vi "PH_SRDG645.get data to modify.vi"(0 "i ref in":refnum<vi>, 3 "ms timeout (10000)":i32=10000, 5 "error in (no error)":errorcluster) -> (14 "i ref out":refnum<vi>, 16 "i attribute":T1={"GUI Refs"={"Delete"=refnum, "Device Errors"=refnum, "Trigger"=refnum, "Default Name"=refnum, "Firmware Revision"=refnum, "Serial Number"=refnum, "Model"=refnum, "Visa resource name"=refnum}, "Service ID Rate"=-1, "Service IDs Channelinfo"=[], "VISA resource name"="", "Device Errors"=[], "Trigger"={"Source"=0, "Rate [Hz]"=1000.0, "Level [V]"=1.0}, "Channels"={"T1"={"Delay [s]"=0.0, "relative to"=0}, "A"={"Delay [s]"=0.0, "relative to"=0}, "B"={"Delay [s]"=0.0, "relative to"=0}, "C"={"Delay [s]"=0.0, "relative to"=0}, "D"={"Delay [s]"=0.0, "relative to"=0}, "E"={"Delay [s]"=0.0, "relative to"=0}, "F"={"Delay [s]"=0.0, "relative to"=0}, "G"={"Delay [s]"=0.0, "relative to"=0}, "H"={"Delay [s]"=0.0, "relative to"=0}}, "GUI Refs Channels"=[], "Outputs"={"AB"={"Level Offset [V]"=0.0, "Amplitue [V]"=0.0, "Polarity"=0}, "CD"={"Level Offset [V]"=0.0, "Amplitue [V]"=0.0, "Polarity"=0}, "EF"={"Level Offset [V]"=0.0, "Amplitue [V]"=0.0, "Polarity"=0}, "GH"={"Level Offset [V]"=0.0, "Amplitue [V]"=0.0, "Polarity"=0}, "T0"={"Level Offset [V]"=0.0, "Amplitue [V]"=0.0, "Polarity"=0}}, "GUI Refs Outputs"=[], "Serial Number"="", "Firmweare Revision"="", "Model"=""} {"Outputs"."T0"."Polarity" items=["negative", "positive"]; "Outputs"."GH"."Polarity" items=["negative", "positive"]; "Outputs"."EF"."Polarity" items=["negative", "positive"]; "Outputs"."CD"."Polarity" items=["negative", "positive"]; "Outputs"."AB"."Polarity" items=["negative", "positive"]; "Channels"."H"."relative to" items=["T0", "T1", "A", "B", "C", "D", "E", "F", "G", "H"]; "Channels"."H"."Delay [s]" format="%#_12p"; "Channels"."G"."relative to" items=["T0", "T1", "A", "B", "C", "D", "E", "F", "G", "H"]; "Channels"."G"."Delay [s]" format="%#_12p"; "Channels"."F"."relative to" items=["T0", "T1", "A", "B", "C", "D", "E", "F", "G", "H"]; "Channels"."F"."Delay [s]" format="%#_12p"; "Channels"."E"."relative to" items=["T0", "T1", "A", "B", "C", "D", "E", "F", "G", "H"]; "Channels"."E"."Delay [s]" format="%#_12p"; "Channels"."D"."relative to" items=["T0", "T1", "A", "B", "C", "D", "E", "F", "G", "H"]; "Channels"."D"."Delay [s]" format="%#_12p"; "Channels"."C"."relative to" items=["T0", "T1", "A", "B", "C", "D", "E", "F", "G", "H"]; "Channels"."C"."Delay [s]" format="%#_12p"; "Channels"."B"."relative to" items=["T0", "T1", "A", "B", "C", "D", "E", "F", "G", "H"]; "Channels"."B"."Delay [s]" format="%#_12p"; "Channels"."A"."relative to" items=["T0", "T1", "A", "B", "C", "D", "E", "F", "G", "H"]; "Channels"."A"."Delay [s]" format="%#_12p"; "Channels"."T1"."relative to" items=["T0", "T1", "A", "B", "C", "D", "E", "F", "G", "H"]; "Channels"."T1"."Delay [s]" format="%#_12p"; "Trigger"."Rate [Hz]" format="%#_9p"; "Trigger"."Source" items=["Internal", "External rising edge", "External falling edge", "Single shot external rising edges", "Single shot external falling edges", "Single shot", "Line"]}, 17 "timed out":bool, 19 "error out":errorcluster)   [LabVIEW 2014, in "PH_SRDG645.lvlib"]
doc: "Reads the attribute data of the object after the access to the data has been locked by the \"acquire\" method. If the attribute data has been locked already, this methods waits until the attribute data is unlocked or there is a timeout.\n\nThe attribute data must be unlocked using the methods \"release\" or \"set modified data\".\n\nLicense Agreement for this software:\n\nCopyright (C)\nGesellschaft für Schwerionenforschung, GSI\nPlanckstr. 1\n64291 Darmstadt\nGermany\n\nContact: D.Beck@gsi.de \n\nThis program is free software; you can redistribute it and/or modify it under the terms of the GNU General Public License as published by the Free Software Foundation; either version 2 of the license, or (at your option) any later version.\n\nThis program is distributed in the hope that it will be useful, but WITHOUT ANY WARRANTY; without even the implied warranty of MERCHANTABILITY or FITNESS FOR A PARTICULAR PURPOSE. See the GNU General License for more details (http://www.gnu.org).\n\nGesellschaft für Schwerionenforschung, GSI\nPlanckstr. 1, 64291 Darmstadt, Germany\nFor all questions and ideas contact: M.Richter@gsi.de, H.Brand@gsi.de or D.Beck@gsi.de.\nLast update: 17-JUN-2004"
uses:
  PH_SRDG645.lvlib
  PH_SRDG645.i attribute.ctl
  PH_SRDG645.Trigger.ctl
  PH_SRDG645.Channel Settings.ctl
  CS_Core/CSObj/CSObj.lvlib
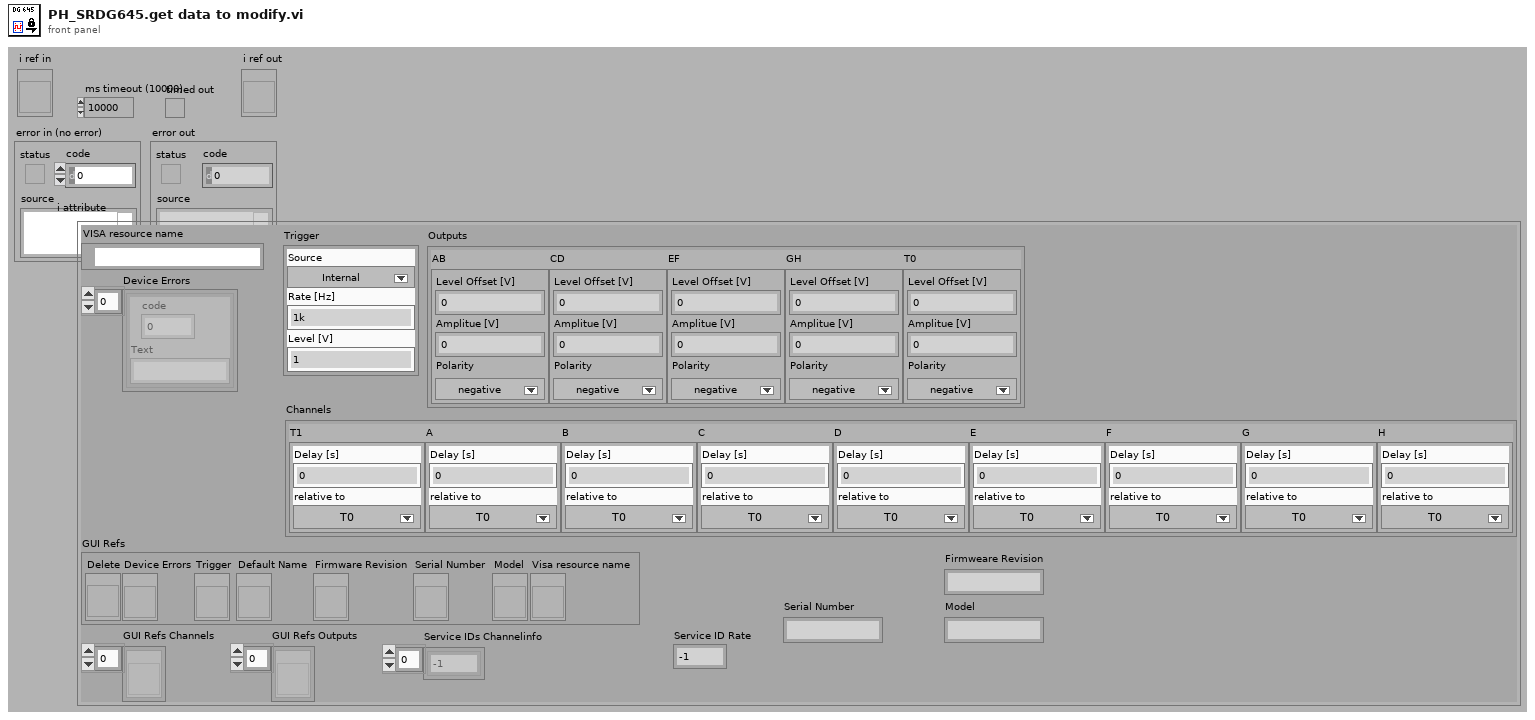
[diagram p1: front panel]
types:
  T1 = typedef "PH_SRDG645.lvlib/PH_SRDG645.i attribute.ctl" = cluster{"GUI Refs":cluster{"Delete":refnum<vi>, "Device Errors":refnum<vi>, "Trigger":refnum<vi>, "Default Name":refnum<vi>, "Firmware Revision":refnum<vi>, "Serial Number":refnum<vi>, "Model":refnum<vi>, "Visa resource name":refnum<vi>}, "Service ID Rate":i32, "Service IDs Channelinfo":i32[], "VISA resource name":refnum<visa-resource-name>, "Device Errors":cluster{"code":i32, "Text":string}[], "Trigger":T2, "Channels":cluster{"T1":T3, "A":T3, "B":T3, "C":T3, "D":T3, "E":T3, "F":T3, "G":T3, "H":T3}, "GUI Refs Channels":refnum<vi>[], "Outputs":cluster{"AB":cluster{"Level Offset [V]":dbl, "Amplitue [V]":dbl, "Polarity":i32}, "CD":cluster{"Level Offset [V]":dbl, "Amplitue [V]":dbl, "Polarity":i32}, "EF":cluster{"Level Offset [V]":dbl, "Amplitue [V]":dbl, "Polarity":i32}, "GH":cluster{"Level Offset [V]":dbl, "Amplitue [V]":dbl, "Polarity":i32}, "T0":cluster{"Level Offset [V]":dbl, "Amplitue [V]":dbl, "Polarity":i32}}, "GUI Refs Outputs":refnum<vi>[], "Serial Number":string, "Firmweare Revision":string, "Model":string}
  T2 = typedef "PH_SRDG645.lvlib/PH_SRDG645.Trigger.ctl" = cluster{"Source":i32, "Rate [Hz]":dbl, "Level [V]":dbl}
  T3 = typedef "PH_SRDG645.lvlib/PH_SRDG645.Channel Settings.ctl" = cluster{"Delay [s]":dbl, "relative to":i32}
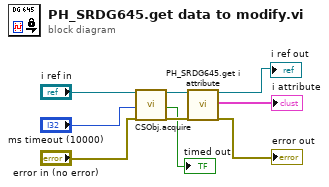
[diagram p0: block diagram]
diagram:
  n1 = call "CSObj.acquire.vi"("i ref in"="i ref in", "ms timeout (10000)"="ms timeout (10000)", "error in (no error)"="error in (no error)") -> ("i ref out"=w8:refnum<vi>, "timed out"=→"timed out":bool, "error out"=w5:errorcluster)  [unwired: 14 in]
  n2 = call "PH_SRDG645.get i attribute.vi"("i ref in"=w8, "error in (no error)"=w5) -> ("i ref out"=→"i ref out":refnum<vi>, "i attribute"=→"i attribute":T1, "error out"=→"error out":errorcluster)  [unwired: 15 in]
